vi "LIDAR_LDS-006.vi"() -> ()   [LabVIEW 2023]
uses:
  <vilib>/Instr/_visa.llb/VISA Configure Serial Port (Instr).vi
panel:
  out "status":bool
  in  "Disconnect":bool
  out "Waveform Graph 2":u16[](graph)
  out "Waveform Graph":dbl[](graph)
  out "XY Graph":cluster{dbl[], dbl[]}(graph)
  out "Frame":T1 {"payload"."#3 Reflexion" format="%.0x"; "payload"."#3 Abstand" format="%.0x"; "CRC" format="%04x"; "Winkel" format="%.0x"}
  in  "Start":bool
  in  "Stop":bool
  in  "Close Button":bool
  in  "Connect":bool
  in  "COM PORT":refnum<visa-resource-name>
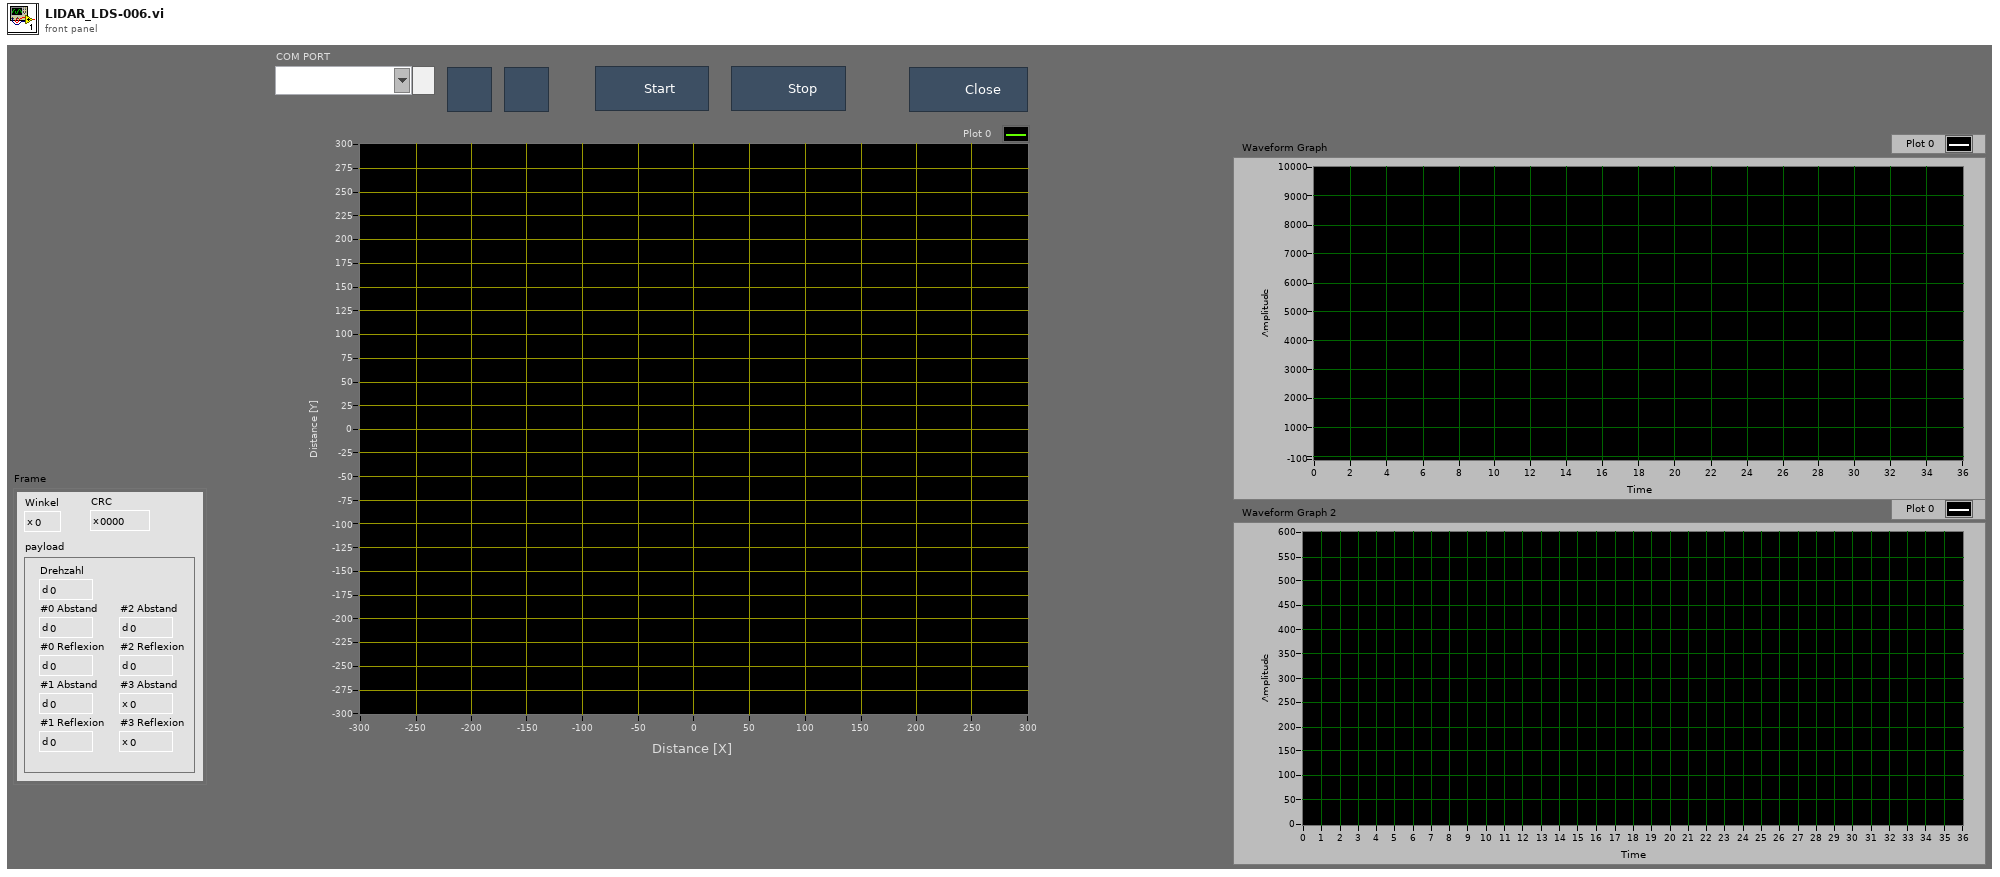
[diagram p1: front panel]
types:
  T1 = cluster{"Winkel":u8, "payload":cluster{"Drehzahl":u16, "#0 Abstand":u16, "#0 Reflexion":u16, "#1 Abstand":u16, "#1 Reflexion":u16, "#2 Abstand":u16, "#2 Reflexion":u16, "#3 Abstand":u16, "#3 Reflexion":u16}, "CRC":u16}
  T2 = enum16{"big-endian, network order", "native, host order", "little-endian"}
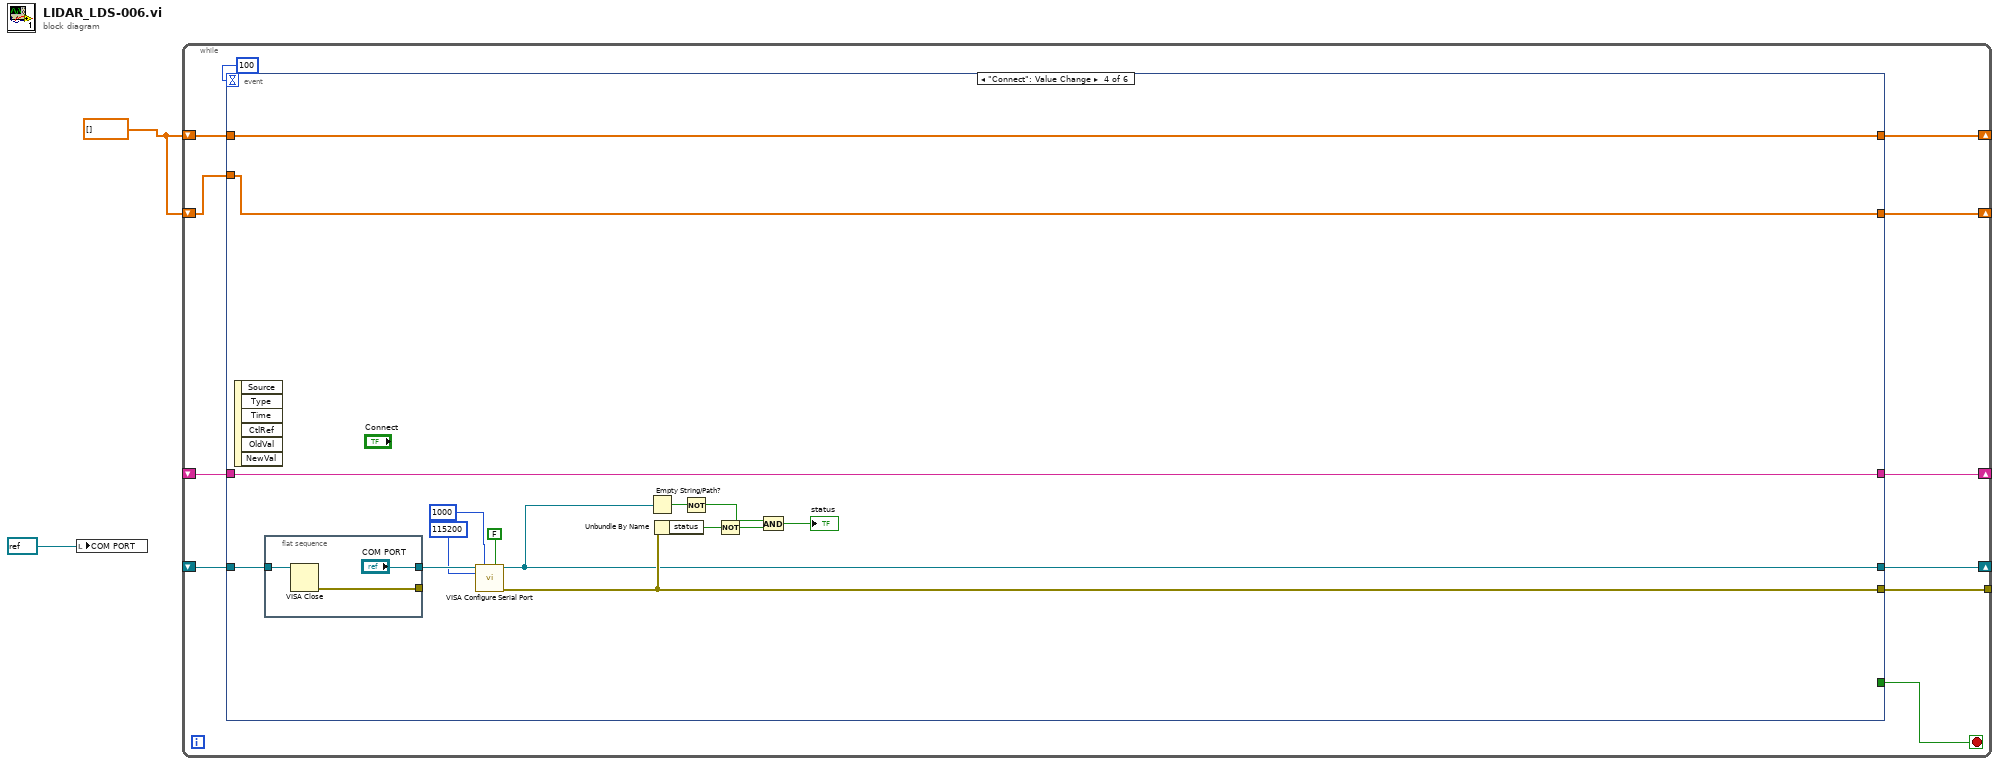
[diagram p0: block diagram]
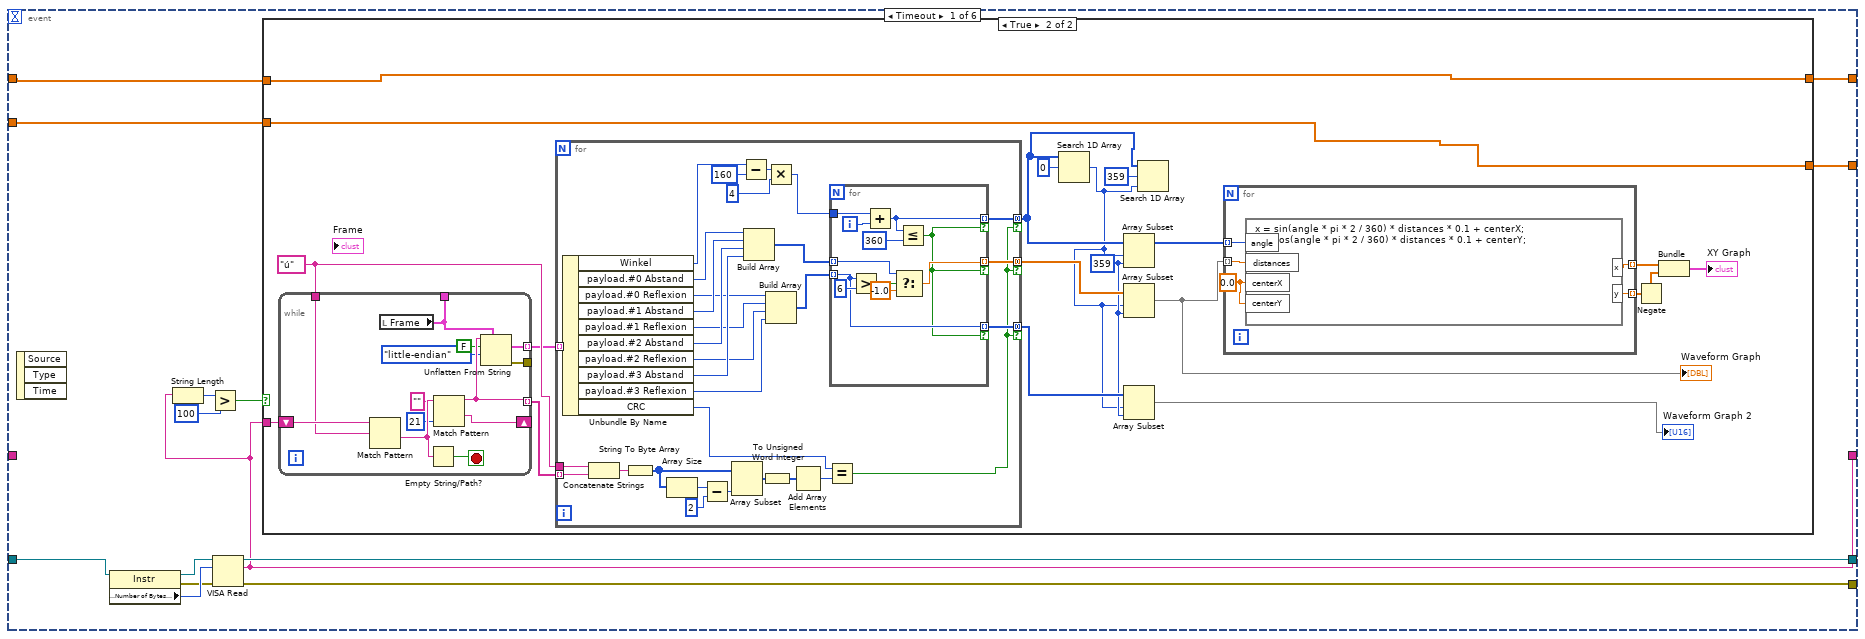
[diagram p2: hidden frame]
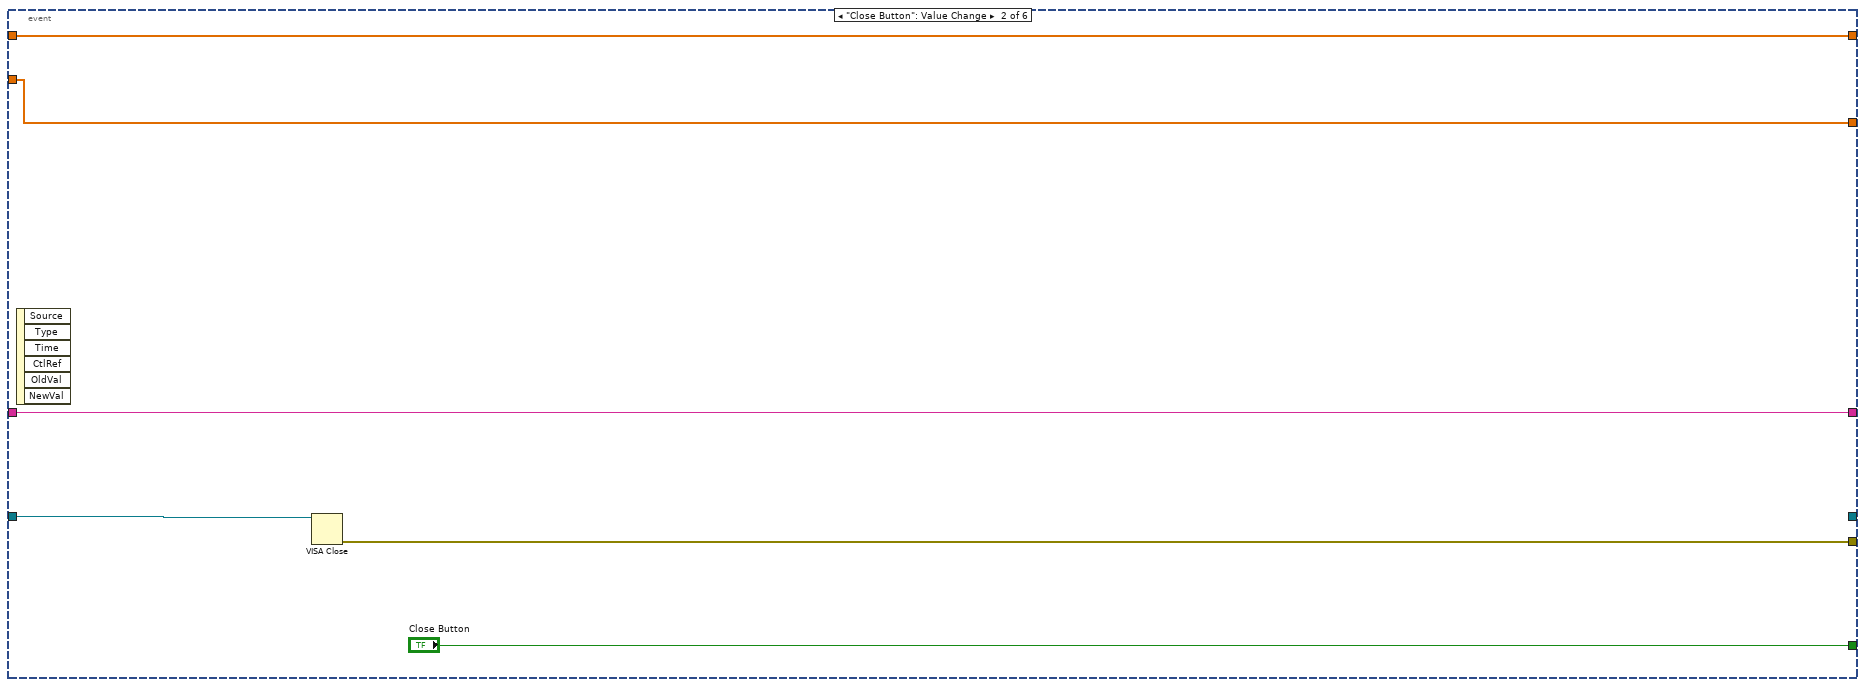
[diagram p4: hidden frame]
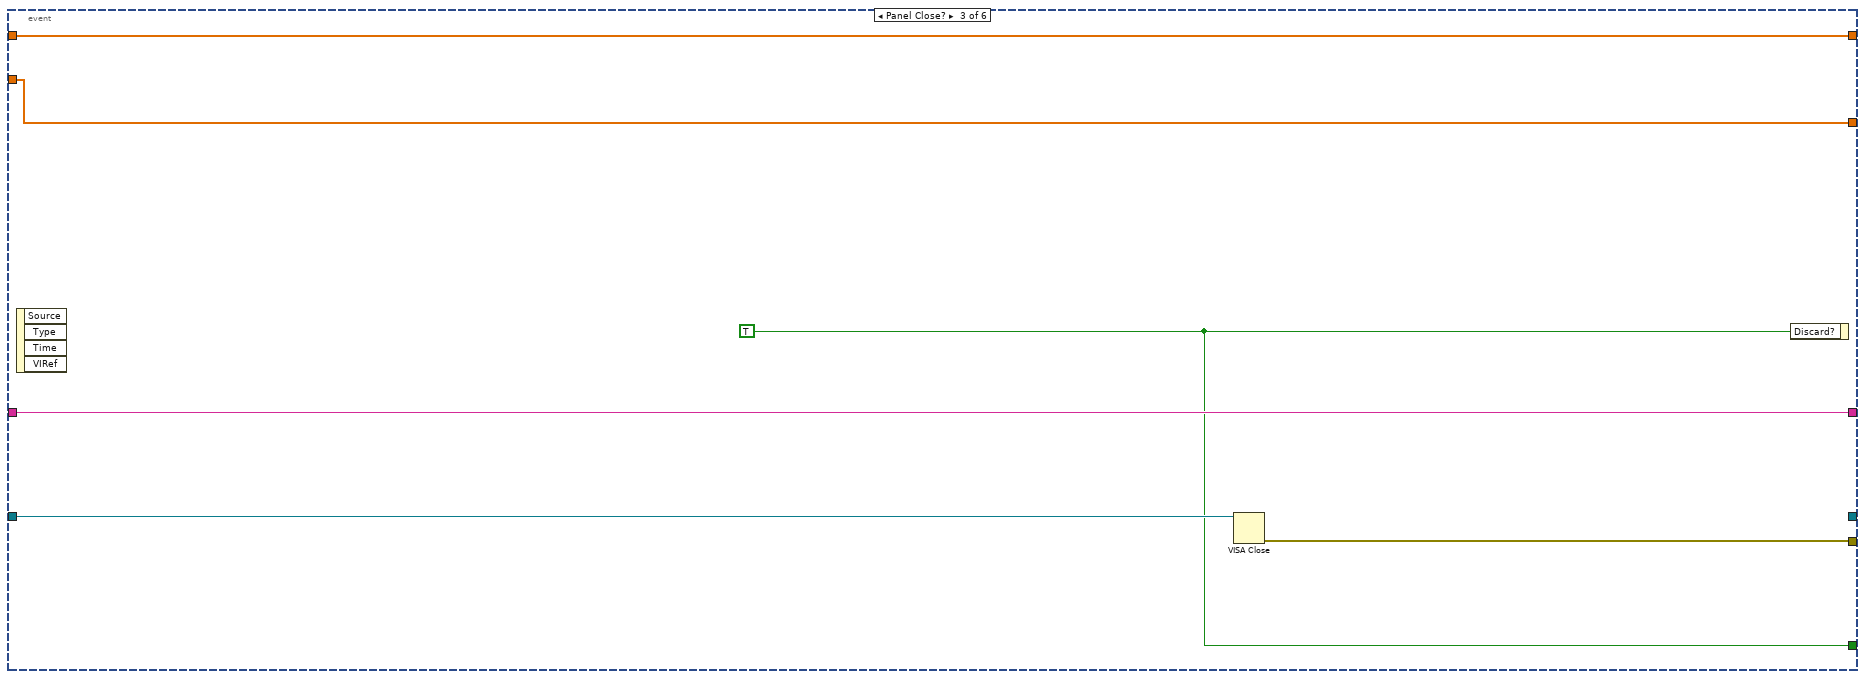
[diagram p5: hidden frame]
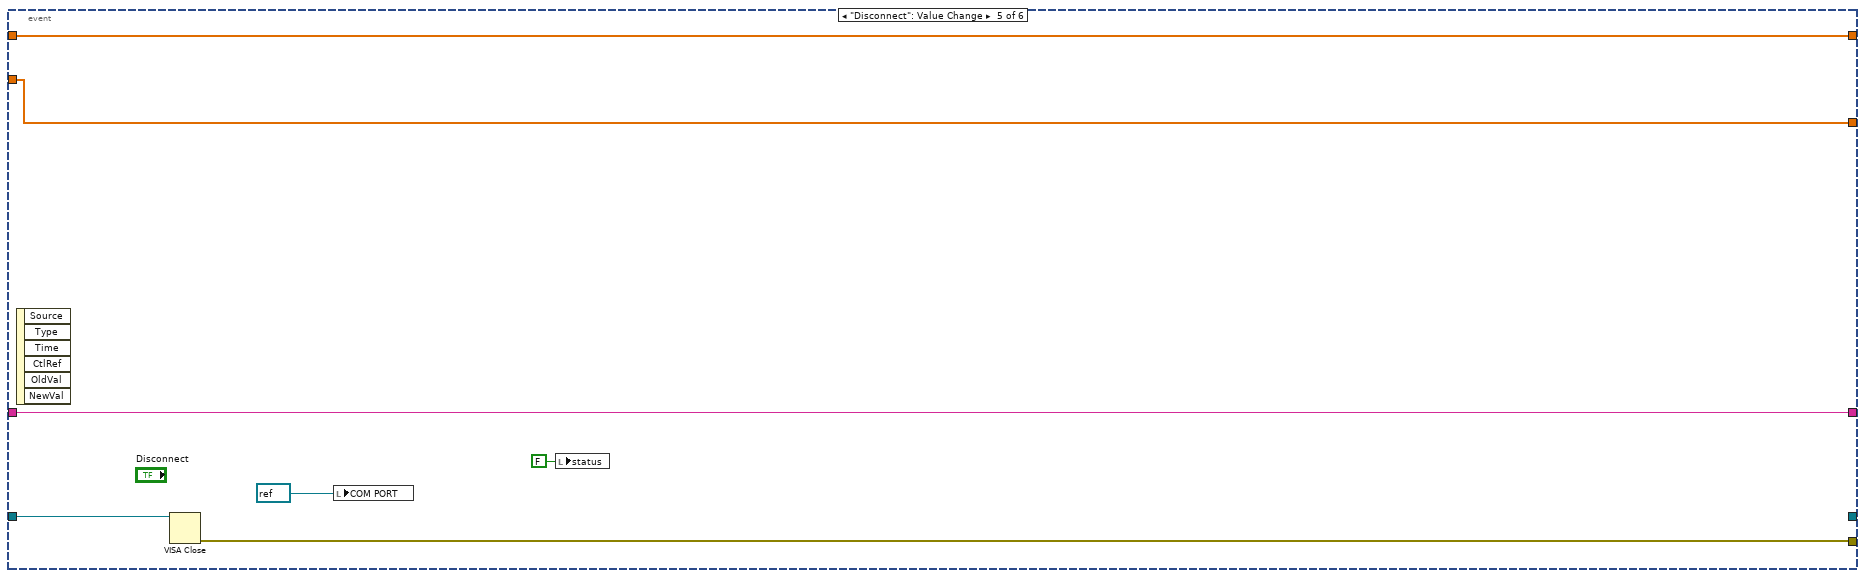
[diagram p6: hidden frame]
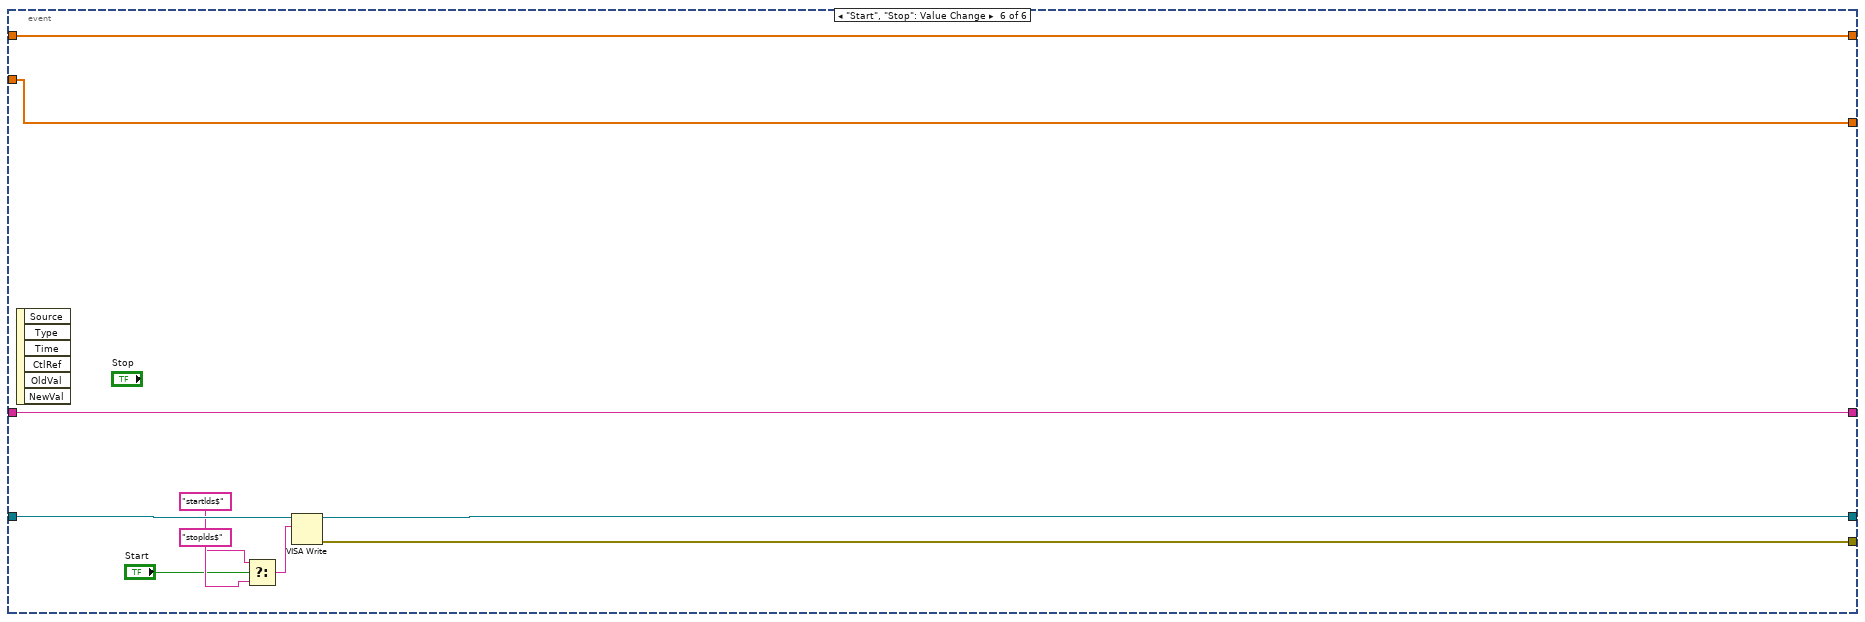
[diagram p7: hidden frame]
diagram:
  w2 = dbl[] []
  n1 = local write "COM PORT"(refnum<visa-resource-name> refnum ("COM PORT")) -> ()
  n2 = while {
    shift-right: [w13] -> _
    shift-left: _ -> [w12]
    tunnel: [w11] -> _
    shift-right: [w9] -> _
    shift-left: _ -> [w8]
    shift-right: [w6] -> _
    shift-left: w2 -> [w5]
    shift-right: [w4] -> _
    shift-left: w2 -> [w3]
    stop <- w7 stop-if-true
    n3 = event shown="[3] \"Connect\": Value Change" {
      selector: _ -> [_ _ _ _ _ _]
      dyn-events: _ -> [_ _ _ _ _ _]
      timeout: 100 ("Numeric 2") -> [_ _ _ _ _ _]
      tunnel: [w27 _ _ w125 _ w154] -> w13
      tunnel: w12 -> [w25 w114 w121 w132 w143 w155]
      tunnel: [w26 w113 w116 w128 w141 w153] -> w11
      tunnel: [w18 w115 w120 w131 w146 w156] -> w9
      tunnel: w8 -> [_ w115 w120 w131 w146 w156]
      tunnel: [_ "Close Button" w117 _ _ _] -> w7
      tunnel: [w17 w110 w119 w130 w145 w148] -> w6
      tunnel: w5 -> [w16 w110 w119 w130 w145 w148]
      tunnel: [w15 w111 w118 w129 w144 w147] -> w4
      tunnel: w3 -> [w14 w111 w118 w129 w144 w147]
      event Timeout {
        n4 = event-data() -> ()  [unwired: 1 in, 3 out]
        n5 = property class="Instr"(reference=w25) -> (reference out=w22:refnum<visa-resource-name>, error out=w23:errorcluster, "Serial Settings:Number of Bytes at Serial Port"=w24:u32)  [unwired: 1 in]
        n6 = VISA Read(VISA resource name=w22, byte count=w24, error in (no error)=w23) -> (VISA resource name out=w27:refnum<visa-resource-name>, read buffer=w18:string, error out=w26:errorcluster)  [unwired: 1 out]
        n7 = String Length(string=w18) -> (length=w21:i32)
        n8 = Greater?(x=w21, y=100) -> (0:w20:bool)
        n9 = case shown="True" w20 {
          tunnel: w18 -> [_ w49]
          tunnel: [w28 w46] -> w17
          tunnel: w16 -> [w28 w46]
          tunnel: [w29 w47] -> w15
          tunnel: w14 -> [w29 w47]
          frame False {
          }
          frame True {
            w32 = "ú" ("regular expression")
            w36 = 359 ("length")
            n10 = while {
              shift-right: [w106] -> _
              shift-left: w49 -> [w109]
              tunnel: [w103] -> w33 mode=indexing
              tunnel: [w97] -> _
              tunnel: [w101] -> _
              tunnel: [w100] -> w31 mode=indexing
              tunnel: w32 -> [w98]
              stop <- w108 stop-if-true
              n11 = Match Pattern(string=w109, regular expression=w98) -> (after substring=w107:string)  [unwired: 1 in, 3 out]
              n12 = local read "Frame"() -> (w97:T1)
              n13 = Empty String/Path?(string/path=w107) -> (empty?=w108:bool)
              n14 = Match Pattern(string=w107, regular expression="", offset (0)=21) -> (before substring=w103:string, after substring=w106:string)  [unwired: 2 out]
              n15 = Unflatten From String(type=w97, binary string=w103, data includes array or string size? (T)=FALSE, byte order (0:big-endian, network order)=T2."little-endian") -> (value=w100:T1, error out=w101:errorcluster)  [unwired: 1 in, 1 out]
            }
            n16 = for {
              tunnel: w31 -> [w85] mode=indexing
              tunnel: [w76] -> w41 mode=concatenating if=w55
              tunnel: [w69] -> w40 mode=concatenating if=w55
              tunnel: [w67] -> w37 mode=concatenating if=w55
              tunnel: w33 -> [w59] mode=indexing
              tunnel: w32 -> [w58]
              n17 = Unbundle By Name(w85) -> ("Winkel"=w84:u8, "payload.#0 Abstand"=w80:u16, "payload.#0 Reflexion"=w74:u16, "payload.#1 Abstand"=w79:u16, "payload.#1 Reflexion"=w73:u16, "payload.#2 Abstand"=w78:u16, "payload.#2 Reflexion"=w72:u16, "payload.#3 Abstand"=w77:u16, "payload.#3 Reflexion"=w71:u16, "CRC"=w56:u16)
              n18 = Concatenate Strings(w58, w59) -> (w66:string)
              n19 = String To Byte Array(string=w66) -> (unsigned byte array=w61:u8[])
              n20 = Array Size(array=w61) -> (size(s)=w62:i32)
              n21 = Subtract(x=w62, y=2) -> (x-y=w63:i32)
              n22 = Array Subset(array=w61, length=w63) -> (w64:u8[])  [unwired: 1 in]
              n23 = Subtract(x=w84, y=u8 160) -> (x-y=w82:u8)
              n24 = Build Array(w80, w79, w78, w77) -> (w68:u16[])
              n25 = To Unsigned Word Integer(number=w64) -> (unsigned 16bit integer=w65:u16[])
              n26 = Multiply(x=w82, y=u16 4) -> (x*y=w75:u16)
              n27 = Build Array(w74, w73, w72, w71) -> (w70:u16[])
              n28 = Add Array Elements(numeric array=w65) -> (sum=w57:u16)
              n29 = Equal?(x=w56, y=w57) -> (x = y?=w55:bool)
              n30 = for {
                tunnel: w75 -> [w95]
                tunnel: w68 -> [w89] mode=indexing
                tunnel: [w94] -> w76 mode=indexing if=w86
                tunnel: w70 -> [w87] mode=indexing
                tunnel: [w88] -> w69 mode=indexing if=w86
                tunnel: [w87] -> w67 mode=indexing if=w86
                i -> [w96]
                n31 = Greater?(x=w87, y=u16 6) -> (0:w91:bool)
                n32 = Add(x=w95, y=w96) -> (x+y=w94:i32)
                n33 = Select(t=w89, s=w91, f=-1.0) -> (s? t:f=w88:dbl)
                n34 = Less Or Equal?(x=w94, y=360) -> (x <= y?=w86:bool)
              }
            }
            n35 = Search 1D Array(1D array=w41, element=0) -> (index of element=w35:i32)  [unwired: 1 in]
            n36 = Array Subset(array=w41, index=w35, length=w36) -> (w39:i32[])
            n37 = Array Subset(array=w40, index=w35, length=w36) -> (w38:dbl[])
            "Waveform Graph" <- w38
            n38 = Array Subset(array=w37, index=w35, length=w36) -> (→"Waveform Graph 2":u16[])
            n39 = Search 1D Array(1D array=w41, element=359, start index (0)=w35) -> ()  [unwired: 1 out]
            n40 = for {
              tunnel: [w54] -> w45 mode=indexing
              tunnel: w39 -> [w53] mode=indexing
              tunnel: w38 -> [w52] mode=indexing
              tunnel: [w51] -> w44 mode=indexing
              w50 = 0.0 ("input variable")
              n41 = formula code="x = sin(angle * pi * 2 / 360) * distances * 0.1 + centerX;\ny = cos(angle * pi * 2 / 360) * distances * 0.1 + centerY;"("angle"=w53, "distances"=w52, "centerX"=w50, "centerY"=w50) -> ("x"=w54:dbl, "y"=w51:dbl)
            }
            n42 = Negate(x=w44) -> (-x=w30:dbl[])
            n43 = Bundle(w45, w30) -> (→"XY Graph":cluster{dbl[], dbl[]})  [unwired: 1 in]
          }
        }
      }
      event "Close Button": Value Change {
        n44 = event-data() -> ()  [unwired: 1 in, 6 out]
        n45 = VISA Close(VISA resource name=w114) -> (error out=w113:errorcluster)  [unwired: 1 in]
      }
      event Panel Close? {
        w117 = TRUE ("Discard?")
        n46 = event-data() -> ()  [unwired: 1 in, 4 out]
        n47 = VISA Close(VISA resource name=w121) -> (error out=w116:errorcluster)  [unwired: 1 in]
        n48 = event-data("Discard?"=w117) -> ()  [unwired: 1 in, 1 out]
      }
      event "Connect": Value Change {
        n49 = event-data() -> ()  [unwired: 1 in, 6 out]
        n50 = flat-sequence {
          tunnel: ["COM PORT"] -> w136
          tunnel: w132 -> [w138]
          tunnel: [w137] -> _
          frame #0 {
            n51 = VISA Close(VISA resource name=w138) -> (error out=w137:errorcluster)  [unwired: 1 in]
          }
        }
        n52 = call-poly "VISA Configure Serial Port"("VISA resource name"=w136, "timeout (10sec)"=u32 1000, "Enable Termination\nChar (T)"=FALSE ("Enable Termination\nChar (T)"), "baud rate (9600)"=u32 115200) -> ("VISA resource name out"=w125:refnum<visa-resource-name>, "error out"=w128:errorcluster)  [unwired: 10 in]
        n53 = Empty String/Path?(string/path=w125) -> (empty?=w123:bool)
        n54 = Unbundle By Name(w128) -> ("status"=w127:bool)
        n55 = Not(x=w123) -> (.not. x?=w122:bool)
        n56 = Not(x=w127) -> (.not. x?=w126:bool)
        n57 = And(x=w122, y=w126) -> (x .and. y?=→"status":bool)
      }
      event "Disconnect": Value Change {
        n58 = event-data() -> ()  [unwired: 1 in, 6 out]
        n59 = VISA Close(VISA resource name=w143) -> (error out=w141:errorcluster)  [unwired: 1 in]
        n60 = local write "COM PORT"(refnum<visa-resource-name> refnum ("COM PORT")) -> ()
        n61 = local write "status"(FALSE ("status")) -> ()
      }
      event "Start", "Stop": Value Change {
        n62 = event-data() -> ()  [unwired: 1 in, 6 out]
        n63 = Select(t="startlds$" ("write buffer"), s="Start", f="stoplds$" ("write buffer")) -> (s? t:f=w150:string)
        n64 = VISA Write(VISA resource name=w155, write buffer=w150) -> (VISA resource name out=w154:refnum<visa-resource-name>, error out=w153:errorcluster)  [unwired: 1 in, 1 out]
      }
    }
  }
